vi "DAQ.Stop.vi"(8 "error in (no error)":errorcluster, 11 "DAQmx in":refnum<class "DAQmx.lvclass">) -> (0 "error out":errorcluster, 3 "DAQmx out":refnum<class "DAQmx.lvclass">)   [LabVIEW 2016, in "DAQmx.lvclass"]
uses:
  DAQmx.lvclass
  DAQmx.lvclass/DAQmx.ctl
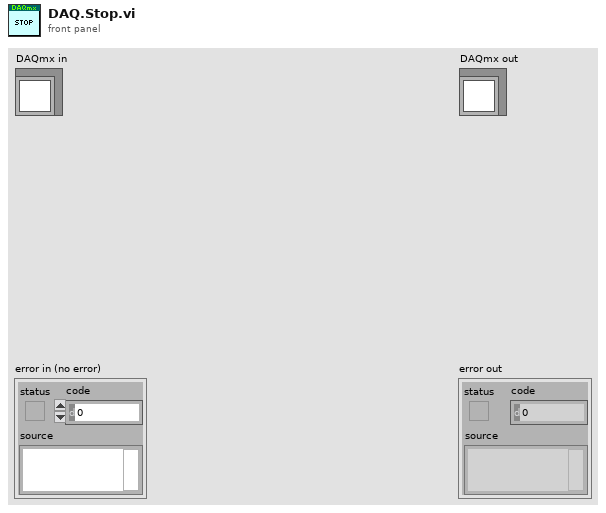
[diagram p1: front panel]
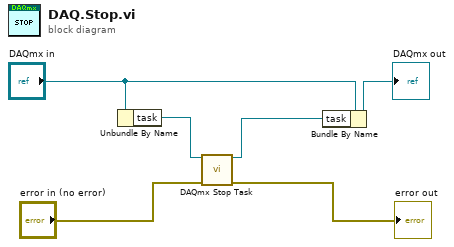
[diagram p0: block diagram]
diagram:
  n1 = Unbundle By Name("DAQmx in") -> ("task"=w3:refnum<k21>)
  n2 = call <vilib>:"DAQmx Stop Task.vi"("task/channels in"=w3, "error in"="error in (no error)") -> ("task out"=w2:refnum<k21>, "error out"=→"error out":errorcluster)  [unwired: 12 in]
  n3 = Bundle By Name(cluster="DAQmx in", "task"=w2) -> (→"DAQmx out":refnum<class "DAQmx.lvclass">)
